vi "rs3 Advanced set depth table control3.vi"(8 "error in (no error)":errorcluster, 10 "Depth Table":T1, 11 "device in":u64) -> (0 "error out 2":errorcluster, 1 "error":u64, 3 "Dev out":u64)   [LabVIEW 2018, in "libRealSense3.lvlib"]
doc: "Sets registers inside the ASIC that affect the depth calculations.\n\nThe depth unit - In microns. By default this is set to 1000, which means the depth map step size is 1mm. The depth range is divided into 65K points. So the max range will then be 65m. \n\ndepth clamp min - limits min depth to this value\ndepth clamp max - limits max depth to this value\ndisparity multiplier - sets a multipler for the displarity output.\ndisparity shift - Normally the D4xx uses a disparity seach range from 0-126, equivalent to seeing objects infinitely far away (disparity 0) to the minZ range nearby (disparity=126). To reduce the minZ it is possible to add a disparity shift. However, false data may then appear if objects are beyond the disparity search range. Generally only use this for near range objects, like objects on a table."
uses:
  libRealSense3.lvlib
  realsense2.dll
panel:
  # "RS3 Adv. Set Depth Table"
  # "(C) 2017 Intel Corp.,  AGJ"
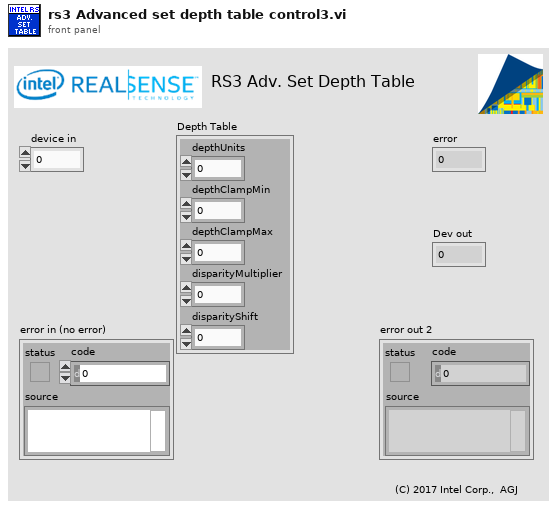
[diagram p1: front panel]
types:
  T1 = cluster{"depthUnits":u32, "depthClampMin":u32, "depthClampMax":u32, "disparityMultiplier":u32, "disparityShift":u32}
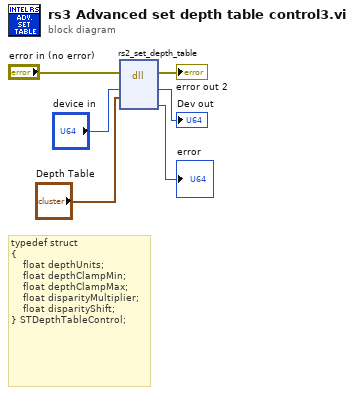
[diagram p0: block diagram]
diagram:
  # "typedef struct\n{\n    float depthUnits;\n    float depthClampMin;\n    float depthClampMax;\n    float disparityMultiplier;\n    float disparityShift;\n} STDepthTableControl;"
  n1 = dll-call lib="C:/Users/aaron.jencks/Documents/GitHub/emerson_seed_object_detection/LabVIEW/Projects/Paul's Video Viewer/Classes/Realsense Cam/realsense_wrapper_api/realsense2.dll" fn="rs2_set_depth_table"(error in="error in (no error)", "device"="device in", "depth table"="Depth Table") -> (error out=→"error out 2":errorcluster, "device"=→"Dev out":u64, "error"=→"error":u64)  [unwired: 5 in, 1 out]
